vi "ValidateAppenderConfigDTO.vi"(8 "error in (no error)":errorcluster, 11 "AppenderConfigDTOin":T1={"id"="", "threshold"="INFO", "filter"={"mode"="Mirror", "levelMin"="INFO", "levelMax"="INFO", "tagPrefix"=""}, "queueBound"=0, "dropPolicy"="DropOldest", "useUTC"=FALSE}) -> (0 "error out":errorcluster, 3 "AppenderConfigDTOout":T1={"id"="", "threshold"="INFO", "filter"={"mode"="mirror", "levelMin"="INFO", "levelMax"="INFO", "tagPrefix"=""}, "queueBound"=0, "dropPolicy"="dropOldest", "useUTC"=FALSE})   [LabVIEW 2026, in "Lumberjack.lvlib"]
uses:
  Lumberjack.lvlib
  TypeDefs/ConfigDTO/AppenderConfigDTO.ctl
  TypeDefs/ConfigDTO/FilterDTO.ctl
  <vilib>/Utility/Data Type/NI_Data Type.lvlib
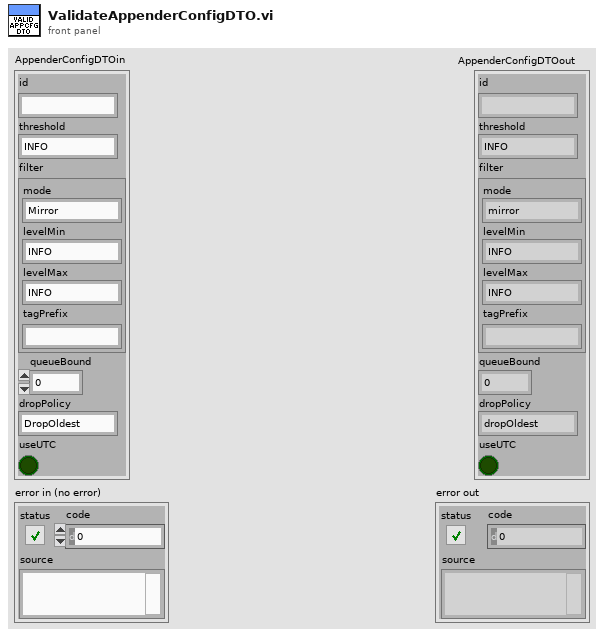
[diagram p1: front panel]
types:
  T1 = typedef "Lumberjack.lvlib/AppenderConfigDTO.ctl" = cluster{"id":string, "threshold":string, "filter":T2, "queueBound":i32, "dropPolicy":string, "useUTC":bool}
  T2 = typedef "Lumberjack.lvlib/FilterDTO.ctl" = cluster{"mode":string, "levelMin":string, "levelMax":string, "tagPrefix":string}
  T3 = typedef "NI_Data Type.lvlib/Data Type.ctl" = enum8{"Invalid Type", "Void", "I8", "I16", "I32", "I64", "U8", "U16", "U32", "U64", "Single Float", "Double Float", "Extended Float", "Single Complex", "Double Complex", "Extended Complex", "Enum U8", "Enum U16", "Enum U32", "Enum U64", "Single Float With Unit", "Double Float With Unit", "Extended Float With Unit", "Single Complex with Unit", "Double Complex with Unit", "Extended Complex with Unit", "Boolean", "String", "Path", "Picture", "Tag", "Array", "Cluster", "Variant", "LV Variant", "Waveform", "Timestamp", "Digital Waveform", "Digital Data", "ExpressData", "Refnum", "External Data", "VI", "Poly VI", "LabVIEW Class Instance", "Fixed Point", "Set Collection", "Map Collection"}
  T4 = typedef "NI_Data Type.lvlib/Type Definition Info.ctl" = cluster{"Name":string, "Timestamp":u32}
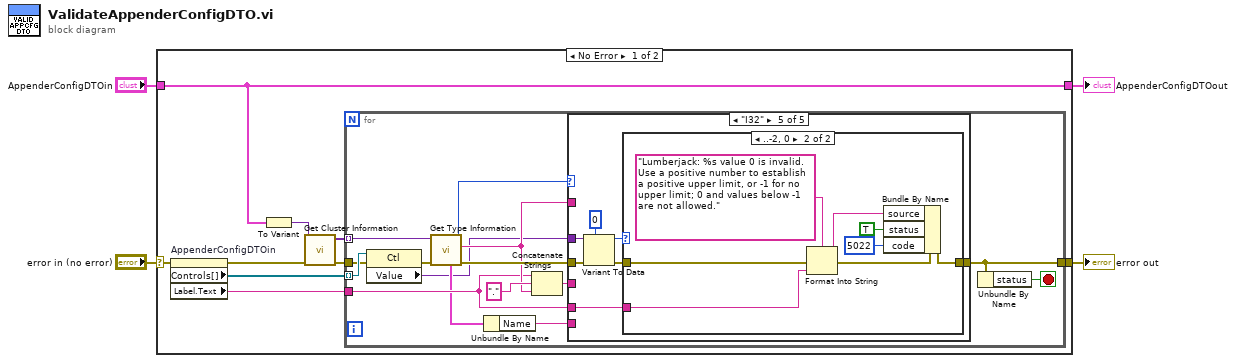
[diagram p0: block diagram]
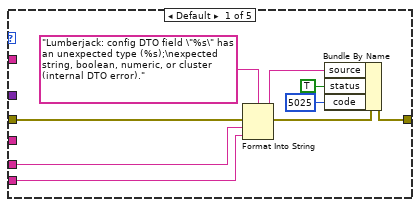
[diagram p2: hidden frame]
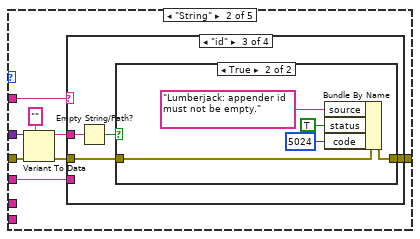
[diagram p3: hidden frame]
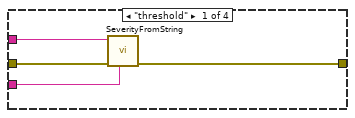
[diagram p4: hidden frame]
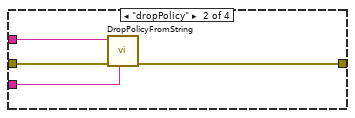
[diagram p5: hidden frame]
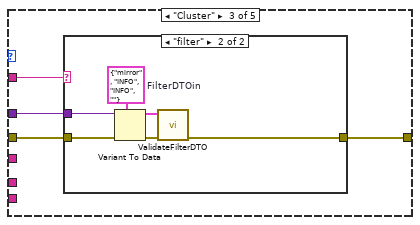
[diagram p8: hidden frame]
diagram:
  n1 = case shown="No Error" "error in (no error)" {
    selector: "error in (no error)" -> [w6 w93]
    tunnel: "AppenderConfigDTOin" -> [w5 w94]
    tunnel: [w7 w93] -> w3
    tunnel: [w5 w94] -> w2
    frame No Error {
      n2 = property on="AppenderConfigDTOin" class="Clust (strict)"(error in=w6) -> (error out=w11:errorcluster, "Controls[]"=w8:refnum<vi>[], "Label.Text"=w9:string)  [unwired: 1 in, 1 out]
      n3 = To Variant(anything=w5) -> (Variant=w10:variant)
      n4 = call <vilib>:"Get Cluster Information.vi"("error in (no error)"=w11, "variant"=w10) -> ("error out"=w12:errorcluster, "cluster elements"=w13:variant[])  [unwired: 8 in]
      n5 = for {
        tunnel: w13 -> [w23] mode=indexing
        tunnel: w12 -> [w16]
        tunnel: w9 -> [w22]
        tunnel: [w19] -> w7
        tunnel: w8 -> [w17] mode=indexing
        stop <- w18 stop-if-true
        n6 = property class="Ctl"(reference=w17, error in=w16) -> (error out=w14:errorcluster, "Value"=w15:variant)  [unwired: 1 out]
        n7 = call <vilib>:"Get Type Information.vi"("error in (no error)"=w14, "variant"=w23) -> ("error out"=w27:errorcluster, "name"=w24:string, "type"=w25:T3, "type definition info"=w21:T4)  [unwired: 5 in, 1 out]
        n8 = Unbundle By Name(w21) -> ("Name"=w20:string)
        n9 = Concatenate Strings(w22, "." ("string"), w24) -> (w26:string)
        n10 = case shown="\"I32\"" w25 {
          tunnel: w27 -> [w33 w43 w68 w76 w81]
          tunnel: w26 -> [_ w45 _ _ _]
          tunnel: w24 -> [_ w44 w66 _ _]
          tunnel: w15 -> [_ w41 w67 _ w79]
          tunnel: w22 -> [w34 _ _ _ w82]
          tunnel: [w30 w38 w65 w76 w83] -> w19
          tunnel: w20 -> [w31 _ _ _ _]
          frame Default {
            n11 = Format Into String(format string="Lumberjack: config DTO field \"%s\" has an unexpected type (%s);\nexpected string, boolean, numeric, or cluster (internal DTO error)." ("source"), error in=w33, w34, w31) -> (resulting string=w29:string, error out=w32:errorcluster)  [unwired: 1 in]
            n12 = Bundle By Name(cluster=w32, "source"=w29, "status"=TRUE, "code"=5025) -> (w30:errorcluster)
          }
          frame "String" {
            n13 = Variant To Data(error in=w43, type="", Variant=w41) -> (data=w39:string, error out=w42:errorcluster)
            n14 = case shown="\"id\"" w44 {
              tunnel: w42 -> [w49 w53 w57 w64]
              tunnel: w45 -> [w48 w52 _ _]
              tunnel: w39 -> [w47 w51 w55 _]
              tunnel: [w46 w50 w56 w64] -> w38
              frame "threshold" {
                n15 = call "SeverityFromString.vi"("Context"=w48, "error in (no error)"=w49, "SeverityString"=w47) -> ("error out"=w46:errorcluster)  [unwired: 7 in, 1 out]
              }
              frame "dropPolicy" {
                n16 = call "DropPolicyFromString.vi"("Context"=w52, "error in (no error)"=w53, "DropPolicyString"=w51) -> ("error out"=w50:errorcluster)  [unwired: 7 in, 1 out]
              }
              frame "id" {
                n17 = Empty String/Path?(string/path=w55) -> (empty?=w54:bool)
                n18 = case shown="True" w54 {
                  tunnel: w57 -> [w58 w61]
                  tunnel: [w58 w60] -> w56
                  frame False {
                  }
                  frame True {
                    n19 = Bundle By Name(cluster=w61, "source"="Lumberjack: appender id must not be empty.", "status"=TRUE, "code"=5024) -> (w60:errorcluster)
                  }
                }
              }
              frame Default {
              }
            }
          }
          frame "Cluster" {
            n20 = case shown="\"filter\"" w66 {
              tunnel: w68 -> [w69 w75]
              tunnel: w67 -> [_ w74]
              tunnel: [w69 w70] -> w65
              frame Default {
              }
              frame "filter" {
                w73 = T2 {"mode"="mirror", "levelMin"="INFO", "levelMax"="INFO", "tagPrefix"=""}  # FilterDTOin
                n21 = Variant To Data(error in=w75, type=w73, Variant=w74) -> (data=w71:T2, error out=w72:errorcluster)
                n22 = call "ValidateFilterDTO.vi"("error in (no error)"=w72, "FilterDTOin"=w71) -> ("error out"=w70:errorcluster)  [unwired: 8 in, 1 out]
              }
            }
          }
          frame "Boolean" {
          }
          frame "I32" {
            n23 = Variant To Data(error in=w81, type=0, Variant=w79) -> (data=w77:i32, error out=w80:errorcluster)
            n24 = case shown="..-2, 0" w77 {
              tunnel: [w84 w90] -> w83
              tunnel: w80 -> [w84 w89]
              tunnel: w82 -> [_ w85]
              frame Default {
              }
              frame ..-2, 0 {
                n25 = Format Into String(format string="Lumberjack: %s value 0 is invalid. Use a positive number to establish a positive upper limit, or -1 for no upper limit; 0 and values below -1 are not allowed." ("source"), error in=w89, w85) -> (resulting string=w87:string, error out=w88:errorcluster)  [unwired: 1 in]
                n26 = Bundle By Name(cluster=w88, "source"=w87, "status"=TRUE, "code"=5022) -> (w90:errorcluster)
              }
            }
          }
        }
        n27 = Unbundle By Name(w19) -> ("status"=w18:bool)
      }
    }
    frame Error {
    }
  }
  "error out" <- w3
  "AppenderConfigDTOout" <- w2
